vi "PS.vi"   [LabVIEW 2016, in "xy_utilities.lvlib"]
uses:
  xy_utilities.lvlib
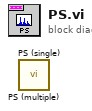
[diagram p0: block diagram]
diagram:
  n1 = call "PS (multiple).vi"() -> ()  [unwired: 9 in, 3 out]
  n2 = call "PS (single).vi"() -> ()  [unwired: 9 in, 3 out]
